vi "dvp Vi Set Output Io Level.vi"(9 "OutputIoLevel":bool, 10 "outputIo":u32(ring)=1 items=["OUTPUT_IO_1"=1, "OUTPUT_IO_2"=2, "OUTPUT_IO_3"=3, "OUTPUT_IO_4"=4, "OUTPUT_IO_5"=5, "OUTPUT_IO_6"=6, "OUTPUT_IO_7"=7, "OUTPUT_IO_8"=8], 11 "handle":u32) -> (3 "function return":u32(ring))   [LabVIEW 2018, in "LabViewDVPCamera.lvlib"]
doc: "LabviewDvp2Api dvpStatus dvpViSetOutputIoLevel(dvpHandle handle, dvpOutputIo outputIo, bool OutputIoLevel);"
uses:
  LabViewDVPCamera.lvlib
  LabViewDVPCamera/LabViewDVPCamera.dll
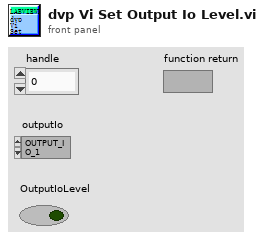
[diagram p1: front panel]
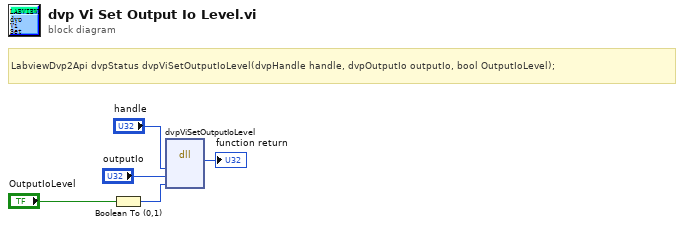
[diagram p0: block diagram]
diagram:
  # "LabviewDvp2Api dvpStatus dvpViSetOutputIoLevel(dvpHandle handle, dvpOutputIo outputIo, bool OutputIoLevel);"
  n1 = Boolean To (0,1)(Boolean="OutputIoLevel") -> (0, 1=w1:i16)
  n2 = dll-call lib="C:/Program Files (x86)/DVP2 Labview cn 64/Sample/LabViewDVPCamera/LabViewDVPCamera.*" fn="dvpViSetOutputIoLevel"("handle"="handle", "outputIo"="outputIo", "OutputIoLevel"=w1) -> (→"function return":u32)  [unwired: 6 in, 2 out]
